vi "FTP_Directory_Listing.vi"() -> ()   [LabVIEW 2014]
uses:
  <vilib>/FTP/NI_FTP.lvlib
panel:
  out "Array":string[](array[string])
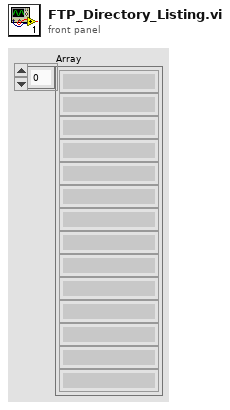
[diagram p1: front panel]
types:
  T1 = typedef "NI_FTP.lvlib/FTP Session.ctl" = refnum<k5>
  T2 = typedef "NI_FTP.lvlib/FTP File Info.ctl" = cluster{"type":enum16{"unknown", "file", "dir", "link"}, "permissions":string, "owner":string, "group":string, "size":i32, "date":string, "name":string, "link name":string}
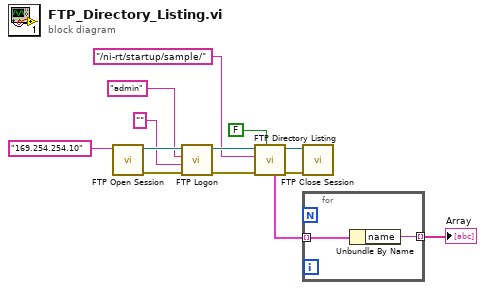
[diagram p0: block diagram]
diagram:
  n1 = call <vilib>:"FTP Open Session.vi"("address"="169.254.254.10") -> ("error out"=w13:errorcluster, "ftp session"=w9:T1)  [unwired: 7 in, 2 out]
  n2 = call <vilib>:"FTP Logon.vi"("error in (no error)"=w13, "password"="", "user"="admin", "ftp session"=w9) -> ("error out"=w12:errorcluster, "ftp session out"=w6:T1)  [unwired: 4 in, 2 out]
  n3 = call <vilib>:"FTP Directory Listing.vi"("active (T)"=FALSE, "error in (no error)"=w12, "directory path"="/ni-rt/startup/sample/", "ftp session"=w6) -> ("error out"=w11:errorcluster, "ftp session out"=w5:T1, "dir list"=w4:T2[])  [unwired: 3 in, 2 out]
  n4 = call <vilib>:"FTP Close Session.vi"("error in (no error)"=w11, "ftp session"=w5) -> ()  [unwired: 6 in, 4 out]
  n5 = for {
    tunnel: w4 -> [w15] mode=indexing
    tunnel: [w14] -> w3 mode=indexing
    n6 = Unbundle By Name(w15) -> ("name"=w14:string)
  }
  "Array" <- w3
